vi "Yolo Swag UDP Test.vi"() -> ()   [LabVIEW 2015]
panel:
  out "error out":errorcluster
  out "data out":string
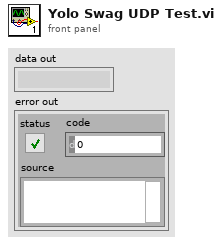
[diagram p1: front panel]
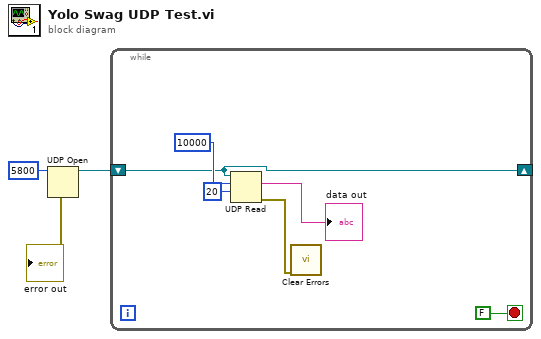
[diagram p0: block diagram]
diagram:
  n1 = UDP Open(11:u16 5800 ("port")) -> (port=w2:refnum<k16>, 0:→"error out":errorcluster)  [unwired: 4 in, 1 out]
  n2 = while {
    shift-right: [w4] -> _
    shift-left: w2 -> [w4]
    stop <- FALSE stop-if-true
    n3 = UDP Read(connection ID=w4, max size (548)=10000, timeout ms (25000)=20) -> (data out=→"data out":string, error out=w5:errorcluster)  [unwired: 1 in, 3 out]
    n4 = call <vilib>:"Clear Errors.vi"("error in (no error)"=w5) -> ()  [unwired: 5 in, 2 out]
  }
